vi "sine.vi"   [LabVIEW 2016]
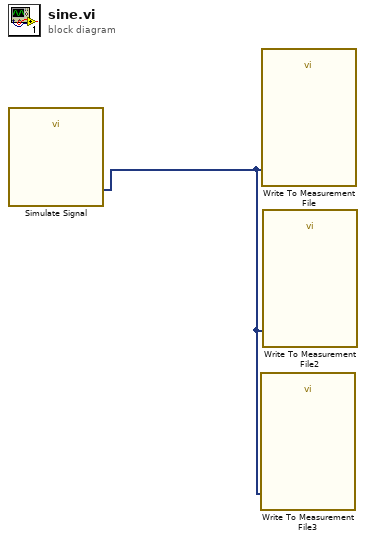
[diagram p0: block diagram]
diagram:
  n1 = call "Simulate Signal"() -> ("Sine"=w1:dynamicdata)  [unwired: 14 in, 1 out]
  n2 = call "Write To Measurement File3"("Signals"=w1) -> ()  [unwired: 16 in, 3 out]
  n3 = call "Write To Measurement File"("Signals"=w1) -> ()  [unwired: 16 in, 3 out]
  n4 = call "Write To Measurement File2"("Signals"=w1) -> ()  [unwired: 16 in, 3 out]
